vi "Run Filter.vi"(8 "error in (no error)":errorcluster, 10 "resource entries in":T1[](array[typedef]) {"FPGA CD Ref" format="%.0x"; "reserver" format="%.0x"}, 11 "RIO Device Filter in":refnum<class "RIO Device Filter.lvclass">) -> (0 "error out":errorcluster, 2 "resource entries out":T1[](array[typedef]) {"FPGA CD Ref" format="%.0x"; "reserver" format="%.0x"})   [LabVIEW 2016, in "RIO Device Filter.lvclass"]
uses:
  RIO Device Filter.lvclass
  Server/viz_entry.ctl
  <vilib>/NI Veristand/Custom Device API/Custom Device Item Ref.ctl
  RIO Device Filter.lvclass/RIO Device Filter.ctl
  FPGA-Addon/Source/Shared/Constants.vi
  <vilib>/NI Veristand/Custom Device API/Get Item Property (String).vi
  <vilib>/NI VeriStand/Custom Device API/Custom Device API.lvlib
  FPGA-Addon/Source/Shared/FPGA Addon Shared.lvlib
  Server/RM.Server.lvlib
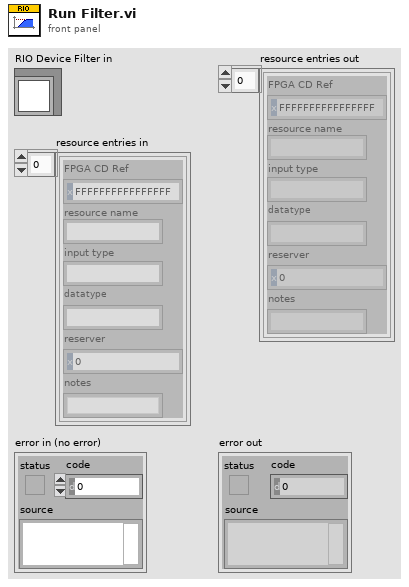
[diagram p1: front panel]
types:
  T1 = typedef "RM.Server.lvlib/viz_entry.ctl" = cluster{"FPGA CD Ref":T2, "resource name":string, "input type":string, "datatype":string, "reserver":T2, "notes":string}
  T2 = typedef "Custom Device API.lvlib/Custom Device Item Ref.ctl" = u64
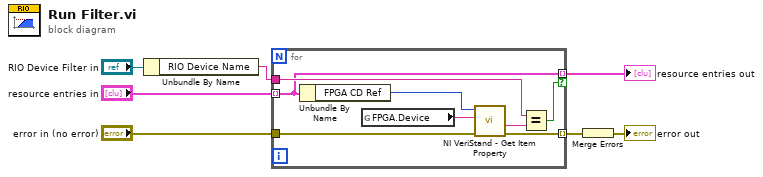
[diagram p0: block diagram]
diagram:
  n1 = Unbundle By Name("RIO Device Filter in") -> ("RIO Device Name"=w5:string)
  n2 = for {
    tunnel: "resource entries in" -> [w11] mode=indexing
    tunnel: w5 -> [w12]
    tunnel: [w11] -> w4 mode=indexing if=w10
    tunnel: "error in (no error)" -> [w9]
    tunnel: [w8] -> w2 mode=indexing
    n3 = Unbundle By Name(w11) -> ("FPGA CD Ref"=w14:T2)
    n4 = global read "Constants.vi" "FPGA.Device"() -> (w15:string)
    n5 = call-poly <vilib>:"NI VeriStand - Get Item Property.vi"("error in (no error)"=w9, "Property Name"=w15, "Item Ref in"=w14) -> ("error out"=w8:errorcluster, "Value"=w13:string)  [unwired: 5 in, 2 out]
    n6 = Equal?(x=w12, y=w13) -> (x = y?=w10:bool)
  }
  "resource entries out" <- w4
  n7 = Merge Errors(w2) -> (→"error out":errorcluster)
